vi "Get Group GObj Refs(冲突时的文件备份2013-05-03 10-36-35).vi"(8 "错误输入（无错误）":errorcluster, 11 "GObj Ref  In":refnum<vi>) -> (0 "错误输出":errorcluster, 1 "Grouped":bool, 2 "Group Member Refs[]":refnum<vi>[](array[refnum]), 3 "GObj Ref Out":refnum<vi>)   [LabVIEW 2012, in "CtrlRef.lvlib"]
uses:
  CtrlRef.lvlib
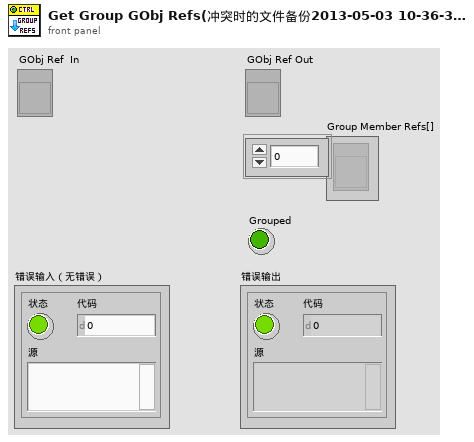
[diagram p1: front panel]
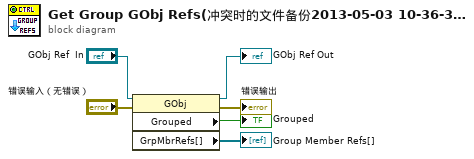
[diagram p0: block diagram]
diagram:
  n1 = property class="GObj"(reference="GObj Ref  In", error in="错误输入（无错误）") -> (reference out=→"GObj Ref Out":refnum<vi>, error out=→"错误输出":errorcluster, "Grouped"=→"Grouped":bool, "GrpMbrRefs[]"=→"Group Member Refs[]":refnum<vi>[])
